vi "drive _initialize.vi"() -> ()   [LabVIEW 2019]
doc: "This example demonstrate how to initailize the drive to use the MoveVelocity, TorqueControl, MoveAbsolute, MoveRealative, MoveAdditive VIs."
uses:
  <vilib>/addons/eal4LabVIEW/ApiLib/Connection control/ealApiConnect_string.vi
  <vilib>/addons/eal4LabVIEW/ApiLib/Connection control/ealApiInitialise_int.vi
  <vilib>/addons/eal4LabVIEW/eal4LabVIEW.lvlib
panel:
  in  "IP address":string="172.17.24.139"
  # "THIAGARAJAR COLLEGE OF ENGINEERING\nDepartment of Mechatronics Engineering"
  # "Introduction"
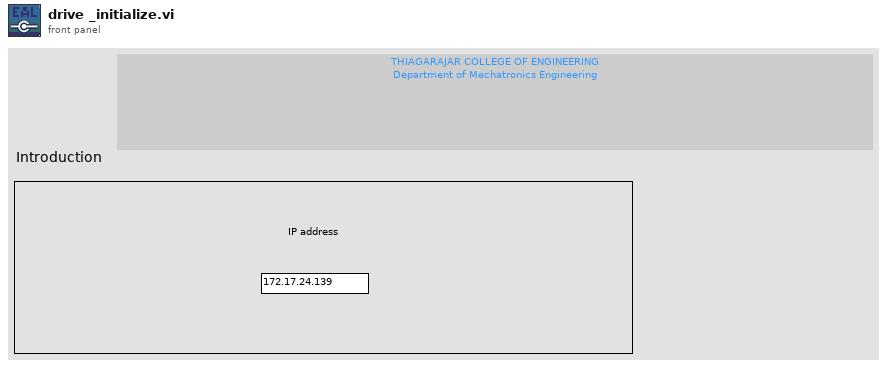
[diagram p1: front panel]
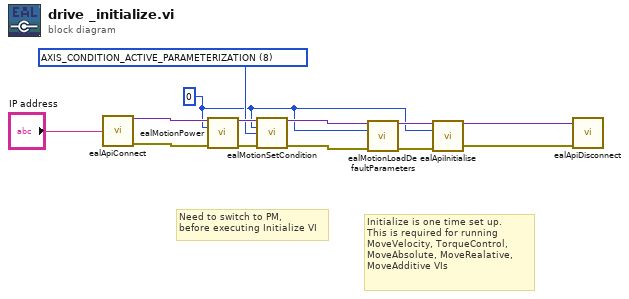
[diagram p0: block diagram]
diagram:
  w6 = 8 items=["AXIS_CONDITION_ACTIVE"=0, "AXIS_CONDITION_PARKING"=1, "AXIS_CONDITION_DEACTIVATED"=2, "AXIS_CONDITION_ACTIVE_DECOUPLED"=4, "AXIS_CONDITION_PARKING_DECOUPLED"=5, "AXIS_CONDITION_DEACTIVATED_DECOUPLED"=6, "AXIS_CONDITION_ACTIVE_PARAMETERIZATION"=8, "AXIS_CONDITION_PARKING_PARAMETERIZATION"=9, "AXIS_CONDITION_DEACTIVATED_PARAMETERIZATION"=10, "AXIS_CONDITION_ACTIVE_DECOUPLED_PARAMETERIZATION"=12, "AXIS_CONDITION_PARKING_DECOUPLED_PARAMETERIZATION"=13, "AXIS_CONDITION_DEACTIVATED_DECOUPLED_PARAMETERIZATION"=14] ("condition")
  w3 = 0 ("slave index")
  # "Need to switch to PM, \nbefore executing Initialize VI"
  # "Initialize is one time set up.\nThis is required for running \nMoveVelocity, TorqueControl, \nMoveAbsolute, MoveRealative, \nMoveAdditive VIs"
  n1 = call-poly <vilib>:"ealApiConnect.vi"("ip address"="IP address") -> ("connection out"=w12:variant, "error out"=w11:errorcluster)  [unwired: 13 in]
  n2 = call <vilib>:"ealMotionPower.vi"("connection in"=w12, "slave index"=w3, "error in (no error)"=w11) -> ("connection out"=w10:variant, "error out"=w9:errorcluster)  [unwired: 11 in]
  n3 = call <vilib>:"ealMotionSetCondition.vi"("connection in"=w10, "slave index"=w3, "condition"=w6, "error in (no error)"=w9) -> ("connection out"=w7:variant, "error out"=w8:errorcluster)  [unwired: 10 in]
  n4 = call <vilib>:"ealMotionLoadDefaultParameters.vi"("connection in"=w7, "slave index"=w3, "error in (no error)"=w8) -> ("connection out"=w5:variant, "error out"=w4:errorcluster)  [unwired: 11 in]
  n5 = call-poly <vilib>:"ealApiInitialise.vi"("connection in"=w5, "slave index"=w3, "error in (no error)"=w4) -> ("connection out"=w2:variant, "error out"=w1:errorcluster)  [unwired: 11 in]
  n6 = call <vilib>:"ealApiDisconnect.vi"("connection in"=w2, "error in (no error)"=w1) -> ()  [unwired: 13 in, 1 out]
